vi "Start Stream.vi"   [LabVIEW 2015, in "niInstr Streaming v1 Host.lvlib"]
uses:
  <instrlib>/_niInstr/Streaming/v1/Host/niInstr Streaming v1 Host.lvlib
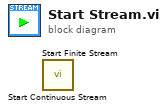
[diagram p0: block diagram]
diagram:
  n1 = call <instrlib>:"Start Continuous Stream.vi"() -> ()  [unwired: 10 in, 2 out]
  n2 = call <instrlib>:"Start Finite Stream.vi"() -> ()  [unwired: 10 in, 2 out]
